vi "Get reference.vi"(8 "Error in":errorcluster, 10 "Vi Path":path, 11 "LV Doc.lvclass":refnum<class "LV Doc.lvclass">) -> (0 "Error Out":errorcluster, 3 "LV Doc.lvclass":refnum<class "LV Doc.lvclass">)   [LabVIEW 2016, in "LV Doc.lvclass"]
doc: "Get reference of given VI."
uses:
  LV Doc.lvclass
  LV Doc.lvclass/LV Doc.ctl
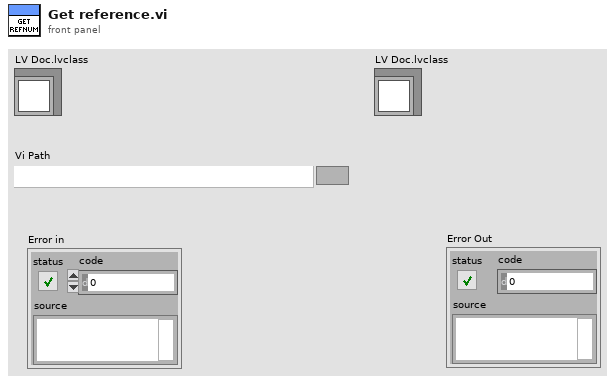
[diagram p1: front panel]
types:
  T1 = enum32{"Invalid", "Standard", "Closed", "Hidden", "Minimized", "Maximized"}
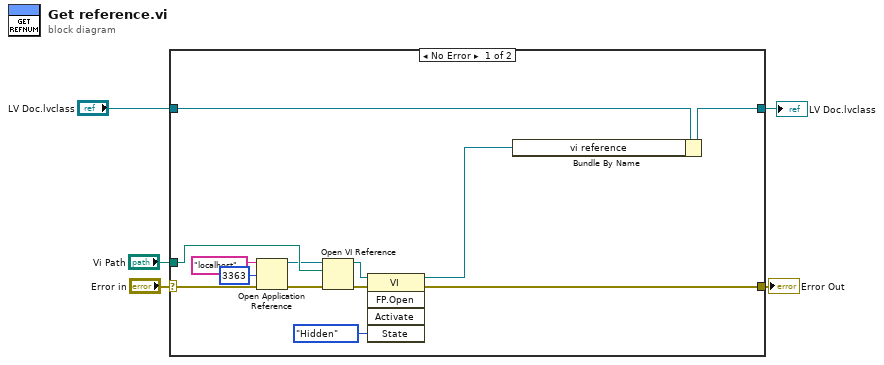
[diagram p0: block diagram]
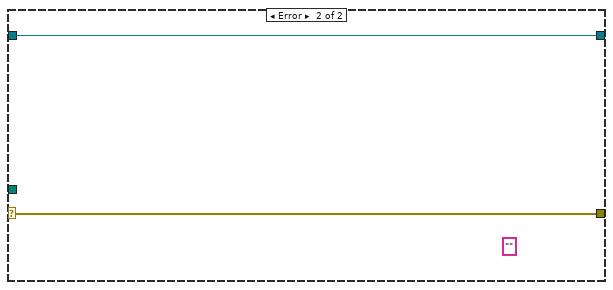
[diagram p2: hidden frame]
diagram:
  n1 = case shown="No Error" "Error in" {
    selector: "Error in" -> [w10 w20]
    tunnel: [w14 w20] -> w4
    tunnel: "Vi Path" -> [w13 _]
    tunnel: "LV Doc.lvclass" -> [w17 w19]
    tunnel: [w16 w19] -> w1
    frame No Error {
      n2 = Open Application Reference(8:w10, 10:u16 3363 ("port number or service name (3363)"), 11:"localhost" ("machine name (\"\":  open local reference)")) -> (0:w9:errorcluster, 3:w8:refnum<vi>)  [unwired: 1 in]
      n3 = Open VI Reference(application reference (local)=w8, vi path=w13, error in (no error)=w9) -> (vi reference=w15:refnum<vi>, error out=w18:errorcluster)  [unwired: 3 in]
      n4 = invoke class="VI" method="FP.Open"(reference=w15, error in=w18, "State"=T1."Hidden") -> (reference out=w12:refnum<vi>, error out=w14:errorcluster)  [unwired: 2 in, 3 out]
      n5 = Bundle By Name(cluster=w17, "vi reference"=w12) -> (w16:refnum<class "LV Doc.lvclass">)
    }
    frame Error {
      (unwired) "" ("Front Panel.Title")
    }
  }
  "Error Out" <- w4
  "LV Doc.lvclass" <- w1
